vi "FPGA_Main.vi"() -> (0 "Chassis Temp History":i16[](array[numeric]), 3 "Chassis Temperature":i16)   [LabVIEW 2020]
uses:
  UIcontrol.ctl
  <vilib>/rvi/interface/RandomDataEmulation/nirviRandomDataOpen.vi
  <vilib>/rvi/interface/common/niFpgaCacheSessionInfoDynamic.vi
  <vilib>/Utility/error.llb/Error Cluster From Error Code.vi
  <vilib>/rvi/errors/niLvFpgaAdjustHostInterfaceError.vi
  <vilib>/rvi/interface/nirviOpenFPGA/nirviOpenFPGA.xnode
  FPGA_Temp.vi
  <vilib>/rvi/interface/nirviReadWriteControl/nirviReadWriteControl.xnode
  NiFpgaLv.dll
  <vilib>/rvi/interface/Simulation/niFpgaSimulationCallBeginRW.vi
panel:
  in  "shutdown?":bool
  in  "save data?":bool
  in  "log?":bool
  in  "shutdown":bool
  in  "save to txt":bool
  in  "grab cRIO data":bool
  # "Remote Panel buttons"
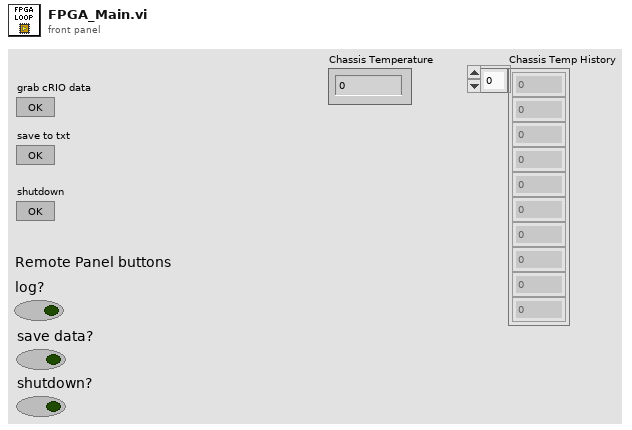
[diagram p1: front panel]
types:
  T1 = typedef "UIcontrol.ctl" = enum16{"Start", "Save Data", "Shutdown"}
  T2 = enum16{"open", "replace", "create", "open or create", "replace or create", "replace or create with confirmation"}
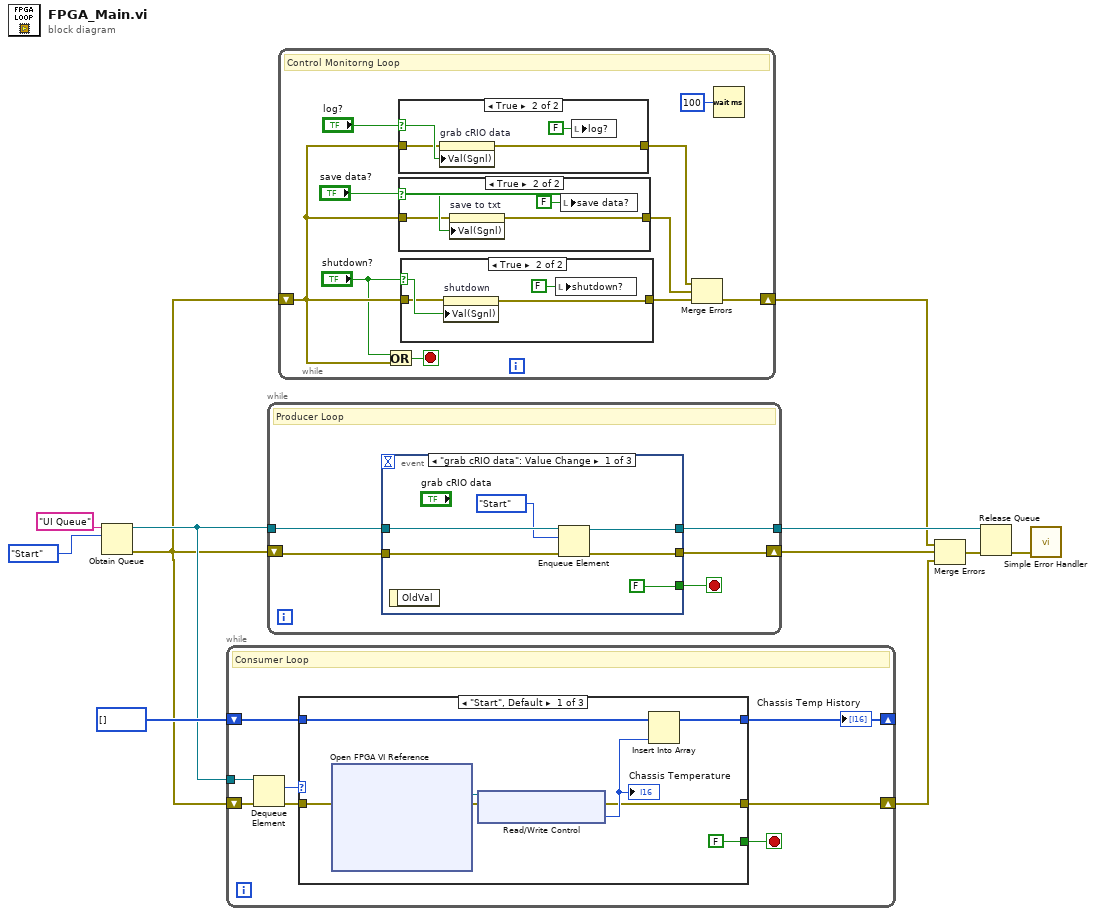
[diagram p0: block diagram]
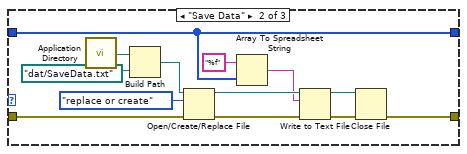
[diagram p5: hidden frame]
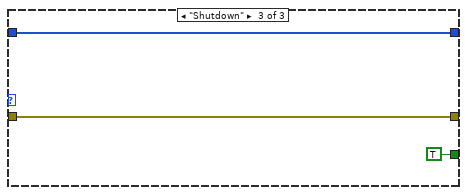
[diagram p6: hidden frame]
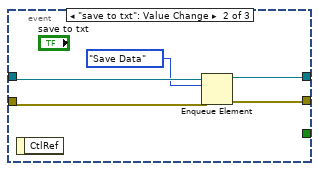
[diagram p7: hidden frame]
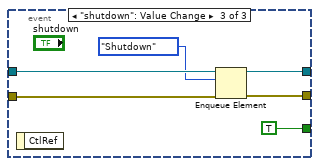
[diagram p8: hidden frame]
diagram:
  n1 = Obtain Queue(name (unnamed)="UI Queue", element data type=UIcontrol."Start") -> (queue out=w5:refnum<queue>, error out=w3:errorcluster)  [unwired: 3 in, 1 out]
  n2 = while {
    tunnel: w5 -> [w19]
    shift-right: [w15] -> _
    shift-left: i16[] [] -> [w14]
    shift-right: [w12] -> w2
    shift-left: w3 -> [w18]
    stop <- w16 stop-if-true
    # "Consumer Loop"
    n3 = Dequeue Element(queue=w19, error in (no error)=w18) -> (element=w17:T1, error out=w13:errorcluster)  [unwired: 1 in, 2 out]
    n4 = case shown="\"Start\", Default" w17 {
      tunnel: [FALSE _ TRUE] -> w16
      tunnel: [w25 w39 w43] -> w15
      tunnel: w14 -> [w24 w39 w43]
      tunnel: w13 -> [w23 w29 w42]
      tunnel: [w20 w28 w42] -> w12
      frame "Start", Default {
        n5 = xnode "Open FPGA VI Reference"("error in"=w23) -> ("FPGA VI Reference Out"=w22:refnum<k20>, "error out"=w21:errorcluster)  [unwired: 1 in]
        n6 = xnode "Read/Write Control"("FPGA VI Reference In"=w22, "error in"=w21) -> ("error out"=w20:errorcluster, "Chassis Temperature"=w26:i16)  [unwired: 1 out]
        "Chassis Temperature" <- w26
        n7 = Insert Into Array(array=w24, new element=w26) -> (w25:i16[])  [unwired: 1 in]
      }
      frame "Save Data" {
        n8 = call <vilib>:"Application Directory.vi"() -> ("Application Directory"=w32:path)
        n9 = Build Path(base path=w32, name or relative path=path "dat/SaveData.txt") -> (appended path=w30:path)
        n10 = Open/Create/Replace File(file path (use dialog)=w30, error in=w29, operation (0:open)=T2."replace or create") -> (refnum out=w37:refnum<file>, error out=w35:errorcluster)  [unwired: 3 in, 1 out]
        n11 = Array To Spreadsheet String(array=w39, 3:"%f" ("format string")) -> (spreadsheet string=w36:string)  [unwired: 1 in]
        n12 = Write to Text File(file (use dialog)=w37, text=w36, error in=w35) -> (refnum out=w34:refnum<file>, error out=w33:errorcluster)  [unwired: 1 in, 1 out]
        n13 = Close File(refnum=w34, error in=w33) -> (error out=w28:errorcluster)  [unwired: 1 out]
      }
      frame "Shutdown" {
      }
    }
    "Chassis Temp History" <- w15
  }
  n14 = while {
    tunnel: w5 -> [w47]
    shift-right: [w45] -> w7
    shift-left: w3 -> [w46]
    tunnel: [w44] -> w9
    stop <- w48 stop-if-true
    # "Producer Loop"
    n15 = event shown="[0] \"grab cRIO data\": Value Change" {
      selector: _ -> [_ _ _]
      dyn-events: _ -> [_ _ _]
      timeout: _ -> [_ _ _]
      tunnel: [FALSE _ TRUE] -> w48
      tunnel: w47 -> [w53 w59 w65]
      tunnel: w46 -> [w52 w57 w64]
      tunnel: [w50 w58 w63] -> w44
      tunnel: [w51 w56 w62] -> w45
      event "grab cRIO data": Value Change {
        n16 = event-data() -> ()  [unwired: 1 in, 1 out]
        n17 = Enqueue Element(queue=w53, element=UIcontrol."Start", error in (no error)=w52) -> (queue out=w50:refnum<queue>, error out=w51:errorcluster)  [unwired: 1 in, 1 out]
      }
      event "save to txt": Value Change {
        n18 = event-data() -> ()  [unwired: 1 in, 1 out]
        n19 = Enqueue Element(queue=w59, element=UIcontrol."Save Data", error in (no error)=w57) -> (queue out=w58:refnum<queue>, error out=w56:errorcluster)  [unwired: 1 in, 1 out]
      }
      event "shutdown": Value Change {
        n20 = event-data() -> ()  [unwired: 1 in, 1 out]
        n21 = Enqueue Element(queue=w65, element=UIcontrol."Shutdown", error in (no error)=w64) -> (queue out=w63:refnum<queue>, error out=w62:errorcluster)  [unwired: 1 in, 1 out]
      }
    }
  }
  n22 = while {
    shift-right: [w71] -> w1
    shift-left: w3 -> [w67]
    stop <- w68 stop-if-true
    # "Control Monitorng Loop"
    n23 = Or(x="shutdown?", y=w67) -> (x .or. y?=w68:bool)
    n24 = case shown="True" "log?" {
      selector: "log?" -> [_ w89]
      tunnel: w67 -> [w86 w88]
      tunnel: [w86 w87] -> w69
      frame False {
      }
      frame True {
        n25 = property on="grab cRIO data" class="Bool (strict)"(error in=w88, "Val(Sgnl)"=w89) -> (error out=w87:errorcluster)  [unwired: 1 in, 1 out]
        n26 = local write "log?"(FALSE ("start cRIO?")) -> ()
      }
    }
    n27 = case shown="True" "save data?" {
      selector: "save data?" -> [_ w84]
      tunnel: w67 -> [w81 w83]
      tunnel: [w81 w82] -> w70
      frame False {
      }
      frame True {
        n28 = property on="save to txt" class="Bool (strict)"(error in=w83, "Val(Sgnl)"=w84) -> (error out=w82:errorcluster)  [unwired: 1 in, 1 out]
        n29 = local write "save data?"(FALSE ("save data?")) -> ()
      }
    }
    n30 = case shown="True" "shutdown?" {
      selector: "shutdown?" -> [_ w80]
      tunnel: w67 -> [w76 w78]
      tunnel: [w76 w77] -> w72
      frame False {
      }
      frame True {
        n31 = property on="shutdown" class="Bool (strict)"(error in=w78, "Val(Sgnl)"=w80) -> (error out=w77:errorcluster)  [unwired: 1 in, 1 out]
        n32 = local write "shutdown?"(FALSE ("shutdown?")) -> ()
      }
    }
    n33 = Merge Errors(w69, w70, w72) -> (w71:errorcluster)
    n34 = Wait (ms)(milliseconds to wait=u32 100) -> ()  [unwired: 1 out]
  }
  n35 = Merge Errors(w1, w7, w2) -> (w8:errorcluster)
  n36 = Release Queue(queue=w9, error in (no error)=w8) -> (error out=w4:errorcluster)  [unwired: 1 in, 2 out]
  n37 = call <vilib>:"Simple Error Handler.vi"("error in (no error)"=w4) -> ()  [unwired: 4 in, 5 out]
